vi "CIPCnewtest.vi"() -> ()   [LabVIEW 2014]
panel:
  out "返り値タイプ 2":string
  out "返り値タイプ":i32
  in  "Connect":bool
  in  "通信設定-Send":T1={"IpAddress"="127.0.0.1", "HostPort"=12000, "SendOrReceive"=2, "ClientPort"=7884, "fps"=100}
  in  "dllパス":path=path "C:/workspace/CIPCSystem/CIPCClient/CIPC_Cpp/CIPCCppDll/Debug/CIPCCppDll.dll"
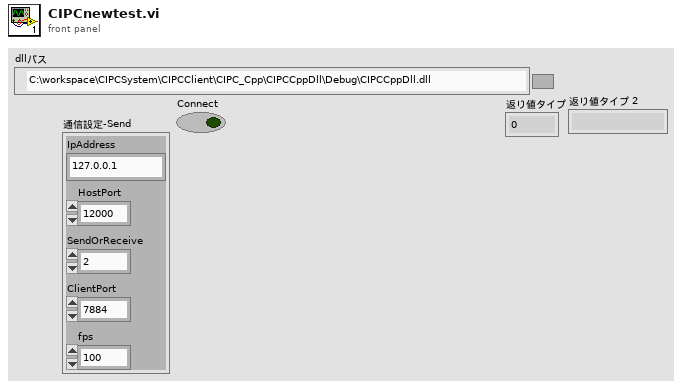
[diagram p1: front panel]
types:
  T1 = cluster{"IpAddress":string, "HostPort":i32, "SendOrReceive":i32, "ClientPort":i32, "fps":i32}
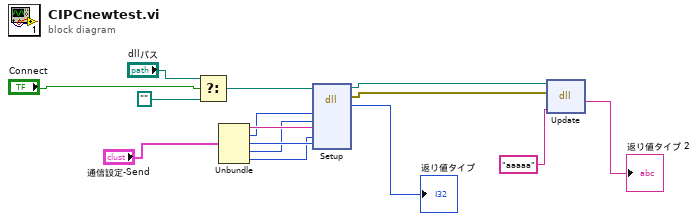
[diagram p0: block diagram]
diagram:
  n1 = Select(t="dllパス", s="Connect", f=path "") -> (s? t:f=w12:path)
  n2 = Unbundle("通信設定-Send") -> ("IpAddress"=w10:string, "HostPort"=w9:i32, "SendOrReceive"=w8:i32, "ClientPort"=w7:i32, "fps"=w6:i32)
  n3 = dll-call lib="C:/workspace/CIPCSystem/CIPCClient/CIPC_Cpp/CIPCCppDll/Debug/CIPCCppDll.dll" fn="Setup"(path in=w12, "serverPort"=w9, "myPort"=w7, "remoteIP"=w10, "fps"=w6, "mode 2s 3r"=w8) -> (path out=w2:path, error out=w1:errorcluster, "返り値タイプ"=→"返り値タイプ":i32)  [unwired: 7 in]
  n4 = dll-call lib="C:/workspace/CIPCSystem/CIPCClient/CIPC_Cpp/CIPCCppDll/Debug/CIPCCppDll.dll" fn="Update"(path in=w2, error in=w1, "serverPort"="aaaaa") -> ("返り値タイプ"=→"返り値タイプ 2":string)  [unwired: 2 in, 2 out]
